vi "Receiver_Monokrom_Mei.vi"() -> ()   [LabVIEW 2018]
uses:
  <vilib>/picture/picture.llb/imagedata.ctl
panel:
  out "new picture 2":picture
  out "image data 2":T1
  out "BER":dbl
  in  "String":string="PENS"
  out "SNR":dbl
  in  "Modulation parameter":T2
  out "created new?":bool
  out "Diagram Constellation":cdb[](graph)
  out "string 2":string
  out "SIG valid?":bool
  out "Frequency offset":dbl
  in  "stop":bool
  out "USRP CoercedParamters":T3={"coerced IQ rate"=100000.0, "coerced carrier frequency"=100000.0, "coerced gain"=0.0} {"coerced gain" format="%#_6f"; "coerced carrier frequency" format="%#_6p"; "coerced IQ rate" format="%#_6p"}
  out "error out":errorcluster
  in  "Trigger level":dbl=0.005 format="%f"
  in  "error in (no error)":errorcluster
  in  "USRP ControledParameters":T4={"active antenna"="RX1", "gain"=20.0, "carrier frequency"=915000000.0, "IQ rate"=1000000.0} {"IQ rate" format="%#_6p"; "carrier frequency" format="%#_6p"; "gain" format="%#_6f"}
  in  "device names":refnum<k15>="192.168.10.2"
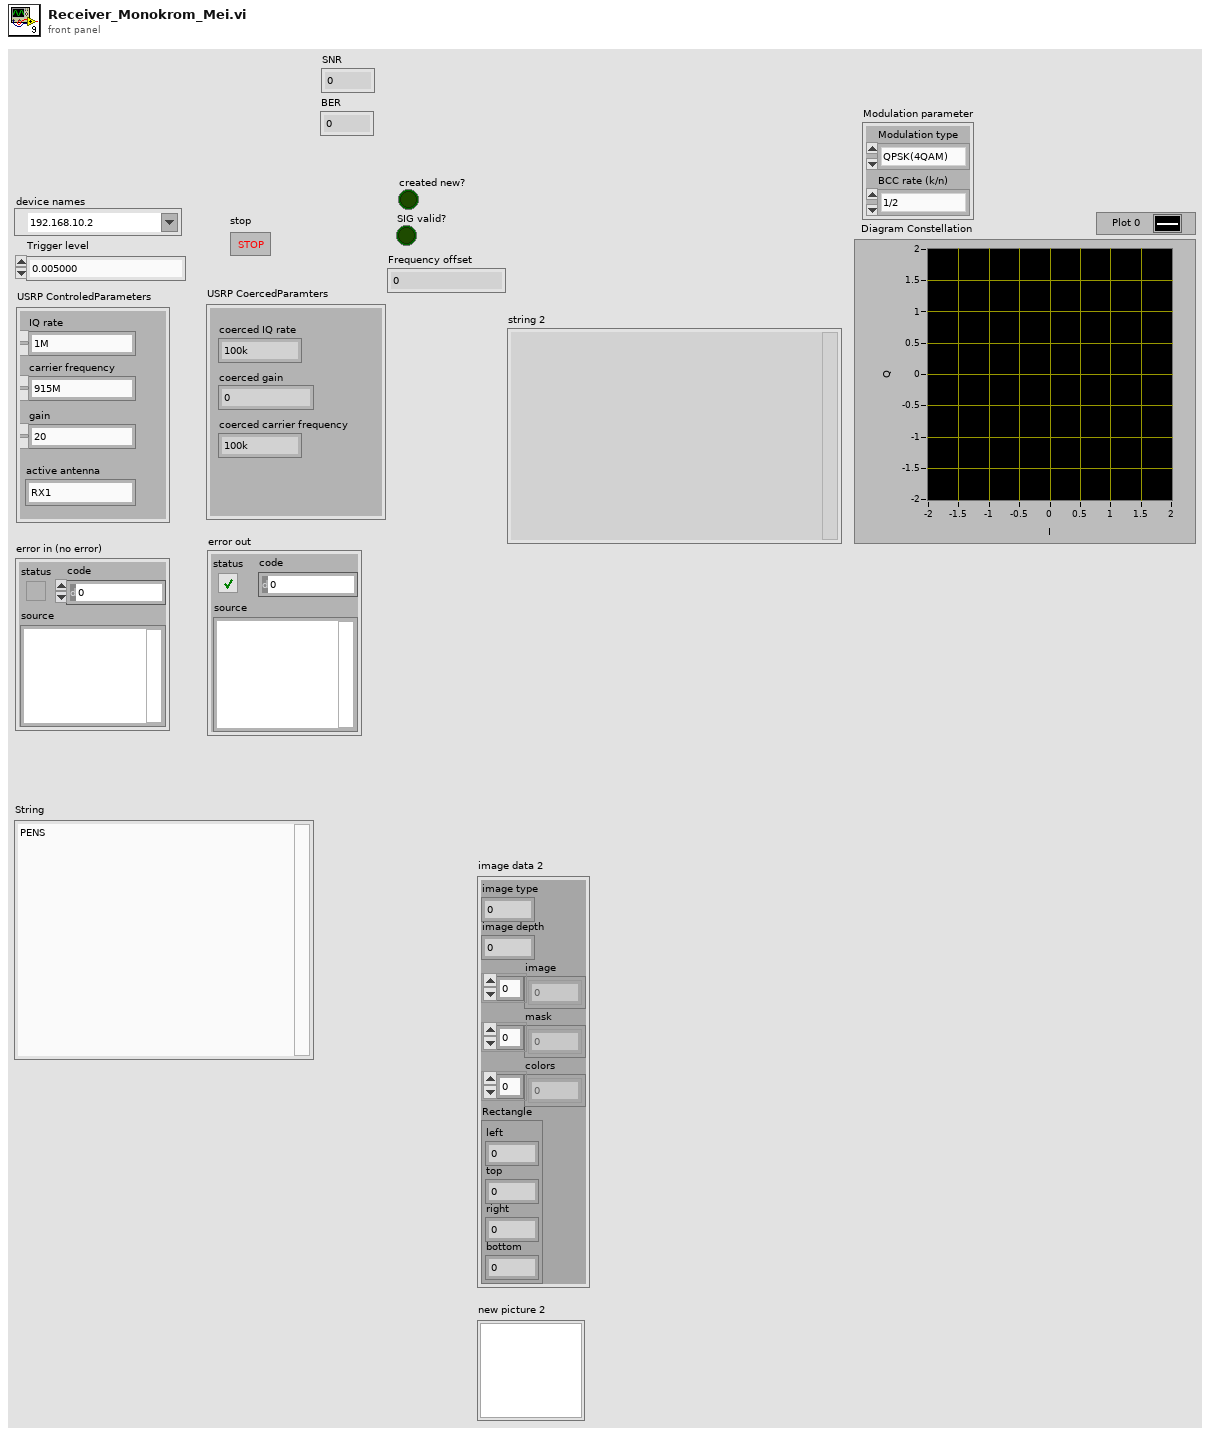
[diagram p1: front panel]
types:
  T1 = typedef "imagedata.ctl" = cluster{"image type":i32, "image depth":i32, "image":u8[], "mask":u8[], "colors":u32[], "Rectangle":cluster{"left":i16, "top":i16, "right":i16, "bottom":i16}}
  T2 = cluster{"Modulation type":enum16{"QPSK(4QAM)", "64QAM", "16QAM", "BPSK"}, "BCC rate (k/n)":enum16{"1/2", "2/3", "3/4"}}
  T3 = cluster{"coerced IQ rate":dbl, "coerced carrier frequency":dbl, "coerced gain":dbl}
  T4 = cluster{"active antenna":string, "gain":dbl, "carrier frequency":dbl, "IQ rate":dbl}
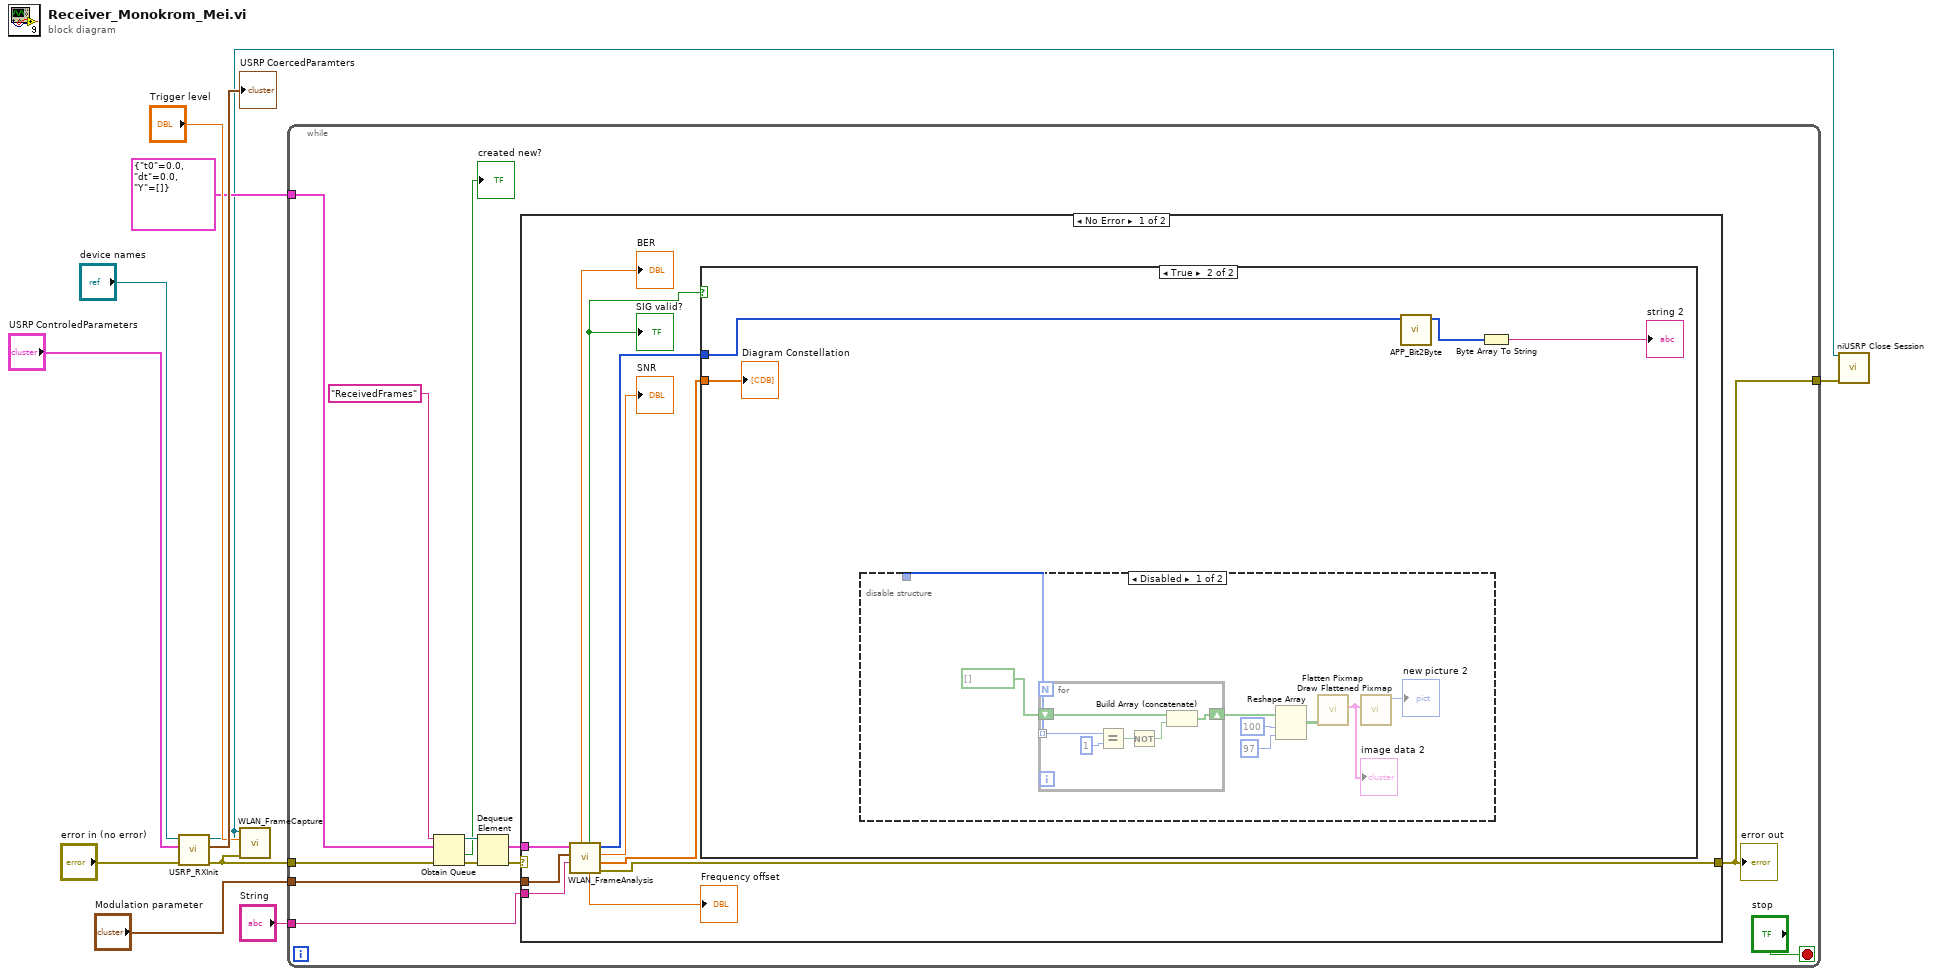
[diagram p0: block diagram]
diagram:
  n1 = call "USRP_RXInit.vi"("device names"="device names", "USRP ControledParameters"="USRP ControledParameters", "error in (no error)"="error in (no error)") -> ("session handle out"=w3:refnum<k15>, "USRP CoercedParamters"=→"USRP CoercedParamters":T3, "error out"=w7:errorcluster)  [unwired: 5 in]
  n2 = call "WLAN_FrameCapture.vi"("error in (no error)"=w7, "Trigger level"="Trigger level", "session handle"=w3) -> ()  [unwired: 8 in]
  n3 = while {
    tunnel: w7 -> [w21]
    tunnel: cluster{"t0":dbl, "dt":dbl, "Y":cdb[]} {"t0"=0.0, "dt"=0.0, "Y"=[]} ("data") -> [w22]
    tunnel: [w14] -> w4
    tunnel: "Modulation parameter" -> [w13]
    tunnel: "String" -> [w12]
    stop <- "stop" stop-if-true
    n4 = Obtain Queue(name (unnamed)="ReceivedFrames", element data type=w22, error in (no error)=w21) -> (queue out=w20:refnum<queue>, created new?=→"created new?":bool, error out=w17:errorcluster)  [unwired: 2 in]
    n5 = Dequeue Element(queue=w20, error in (no error)=w17) -> (element=w18:cluster{"t0":dbl, "dt":dbl, "Y":cdb[]}, error out=w19:errorcluster)  [unwired: 1 in, 2 out]
    n6 = case shown="No Error" w19 {
      selector: w19 -> [_ w52]
      tunnel: w18 -> [w28 _]
      tunnel: [w29 w52] -> w14
      tunnel: w13 -> [w27 _]
      tunnel: w12 -> [w25 _]
      frame No Error {
        n7 = call "WLAN_FrameAnalysis.vi"("String"=w25, "Modulation parameter"=w27, "input cluster"=w28) -> ("error out"=w29:errorcluster, "Constellation"=w30:cdb[], "SNR"=→"SNR":dbl, "output bits"=w31:i8[], "Frequency offset"=→"Frequency offset":dbl, "SIG valid?"=w32:bool, "BER"=→"BER":dbl)  [unwired: 1 in, 1 out]
        "SIG valid?" <- w32
        n8 = case shown="True" w32 {
          tunnel: w31 -> [_ w36]
          tunnel: w30 -> [_ w37]
          frame False {
          }
          frame True {
            n9 = disable-structure shown="Disabled" {
              disable-tunnel: _ -> [w45 _]
              frame Disabled {
                n10 = for {
                  tunnel: w45 -> [w51] mode=indexing
                  shift-right: [w49] -> w38
                  shift-left: bool[] [] -> [w48]
                  n11 = Equal?(x=w51, y=1) -> (x = y?=w47:bool)
                  n12 = Not(x=w47) -> (.not. x?=w46:bool)
                  n13 = Build Array (concatenate)(w48, w46) -> (w49:bool[])
                }
                n14 = Reshape Array(w38, 100 ("dimension size"), 97 ("dimension size")) -> (w41:bool[][])
                n15 = call <vilib>:"Flatten Pixmap.vi"("1-bit pixmap"=w41) -> ("image data"=w40:T1)  [unwired: 10 in]
                "image data 2" <- w40
                n16 = call <vilib>:"Draw Flattened Pixmap.vi"("image data"=w40) -> ("new picture"=→"new picture 2":picture)  [unwired: 8 in]
              }
              frame Enabled {
              }
            }
            n17 = call "APP_Bit2Byte.vi"("input bit stream"=w36) -> ("output byte stream"=w34:u8[])  [unwired: 9 in, 1 out]
            n18 = Byte Array To String(unsigned byte array=w34) -> (string=→"string 2":string)
            "Diagram Constellation" <- w37
          }
        }
      }
      frame Error {
      }
    }
    "error out" <- w14
  }
  n19 = call <instrlib>:"niUSRP Close Session.vi"("session handle"=w3, "error in (no error)"=w4) -> ()  [unwired: 13 in, 1 out]
